vi "Macro Dash.vi"() -> ()   [LabVIEW 2017]
uses:
  VIs/CtrlRefs/GyroTargetInfo.ctl
panel:
  out "CurrentTime":timestamp caption="Robot Time" format="%<%.2X>T"
  in  "Exit":bool
  in  "Tab Control":enum32{"Macro", "Gyro"}(tab)
  out "Boolean":bool
  out "Tank":dbl(slide) caption="Remaining Time" scale=0.0..15.0
  in  "Record Start":bool
  out "Timer":dbl format="%#.1f"
  in  "Record Stop":bool
  in  "Macro Name":string
  in  "Macro delete":bool
  in  "Macros":i32(listbox)
  out "TurnRight":bool
  out "TurnLeft":bool
  out "OnTarget":bool
  out "Gyro":cluster{dbl, dbl}(knob)={0.0, 10.0} scale=0.0..360.0
  # "Tab Controls allow you to have more screens."
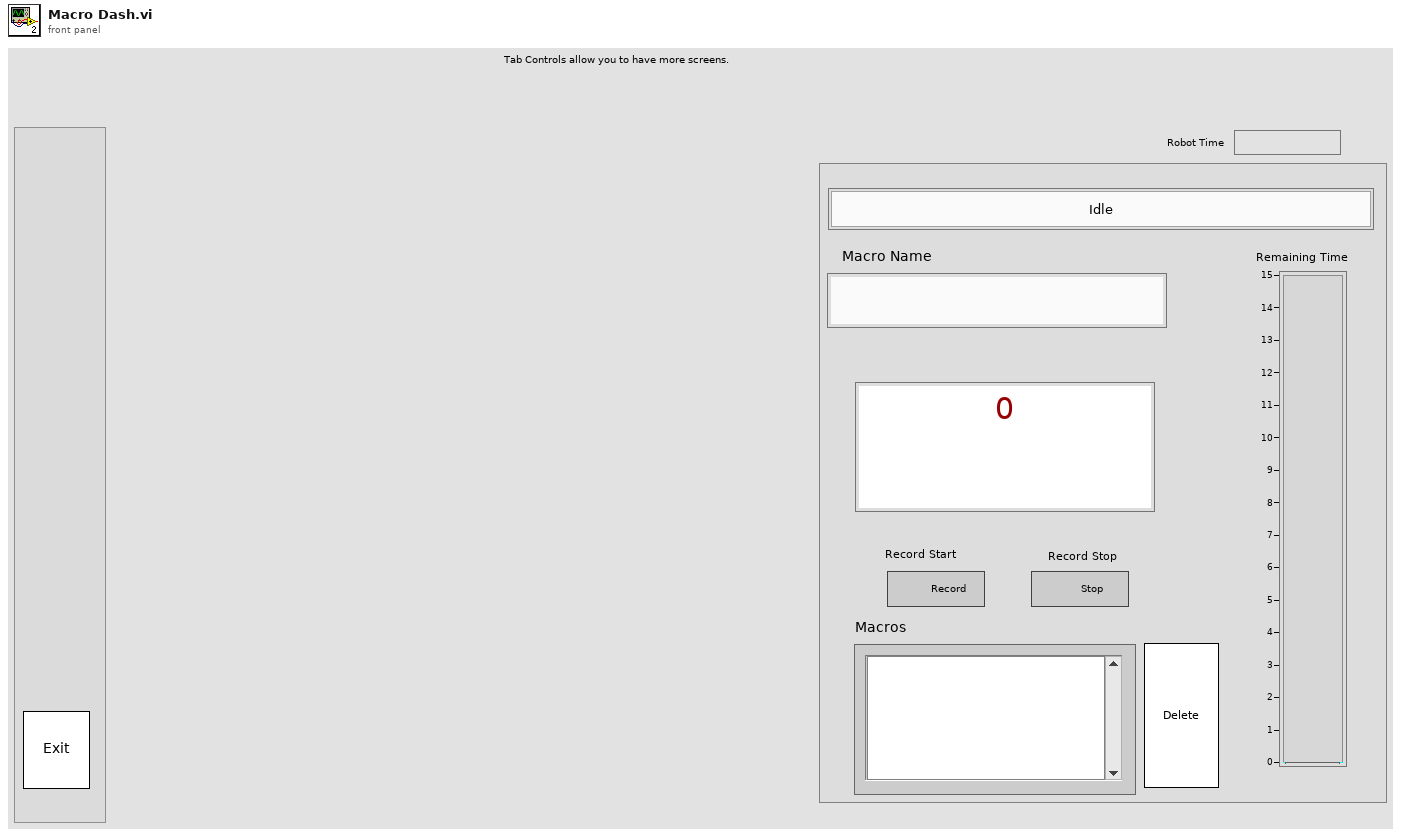
[diagram p1: front panel]
types:
  T1 = typedef "GyroTargetInfo.ctl" = cluster{"Target":dbl, "CurHeading":dbl, "OnTarget":bool, "RotateLeft":bool, "RotateRight":bool, "DegreesToTarget":dbl, "RotDirection":enum16{"Left", "Right", "Stop"}}
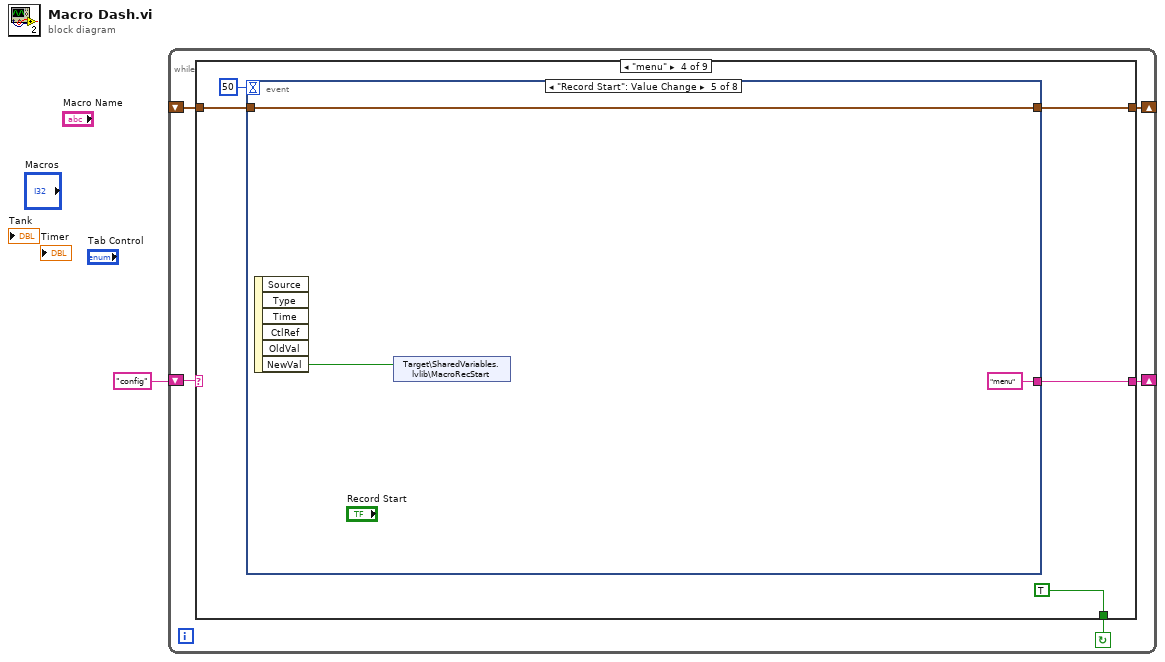
[diagram p0: block diagram]
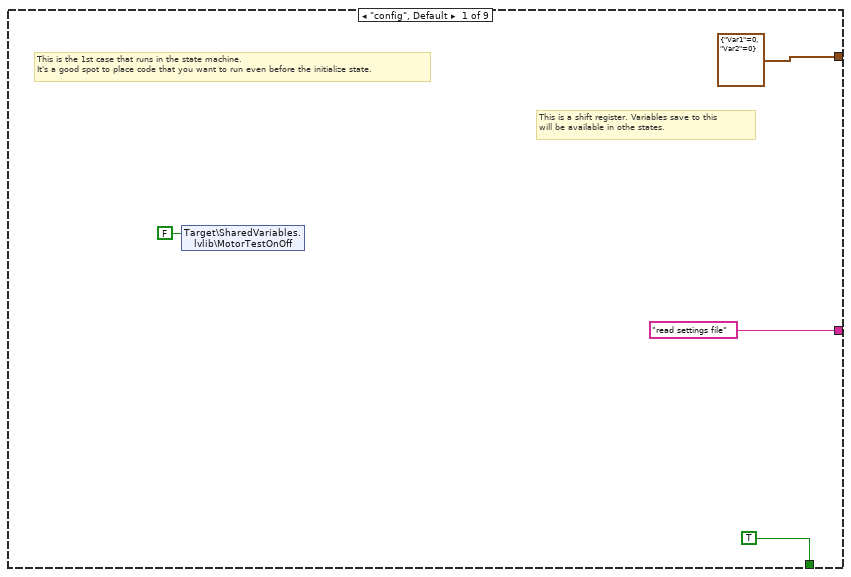
[diagram p2: hidden frame]
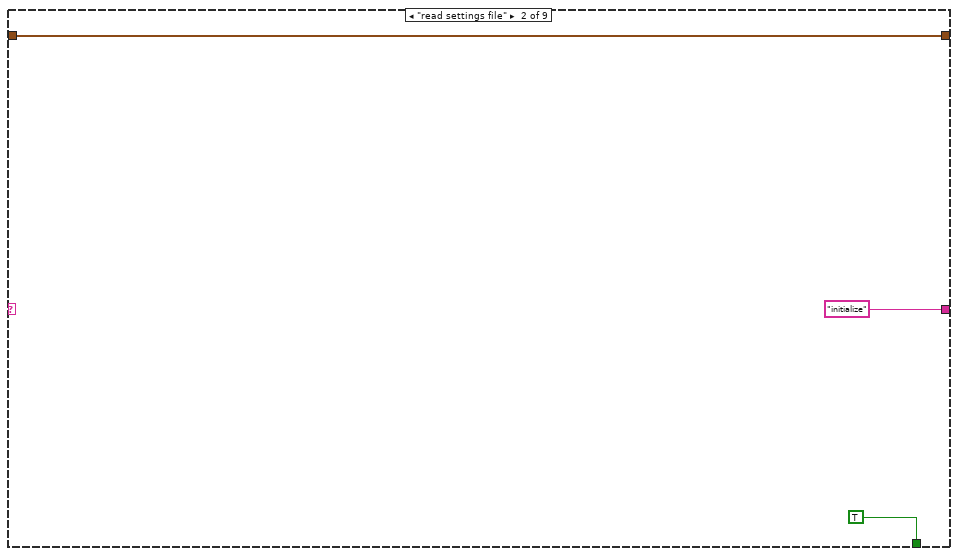
[diagram p3: hidden frame]
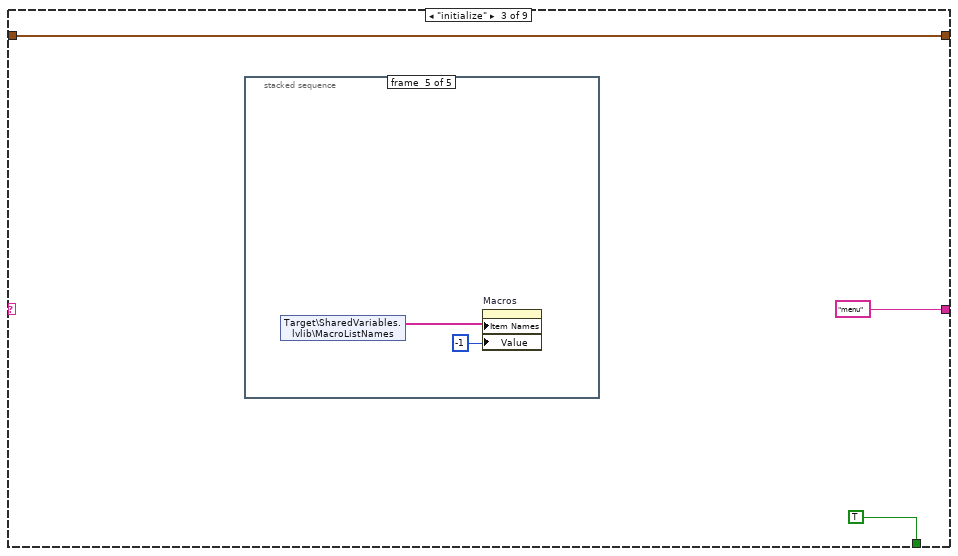
[diagram p4: hidden frame]
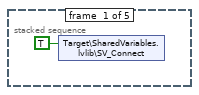
[diagram p5: hidden frame]
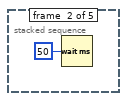
[diagram p6: hidden frame]
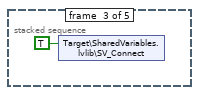
[diagram p7: hidden frame]
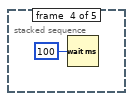
[diagram p8: hidden frame]
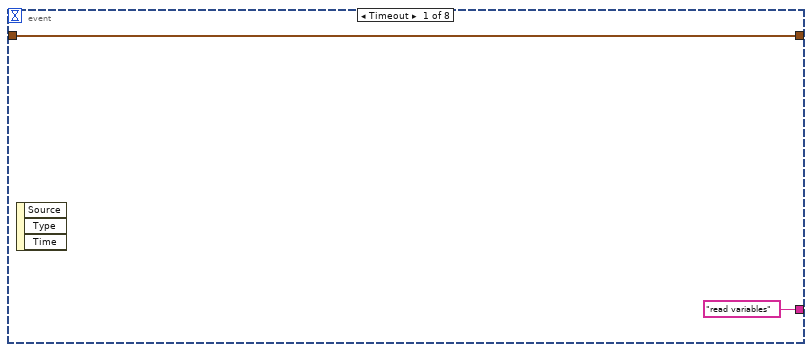
[diagram p9: hidden frame]
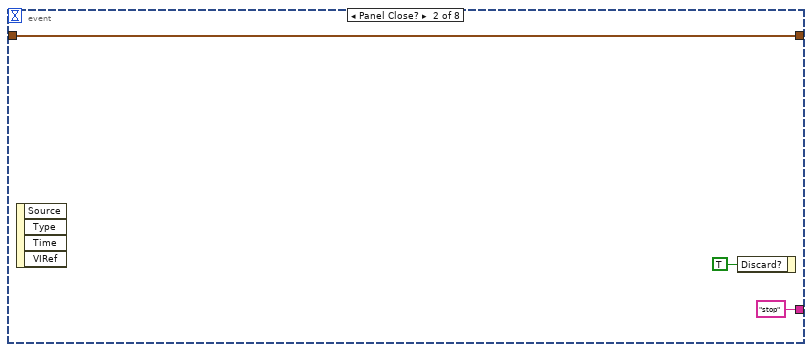
[diagram p10: hidden frame]
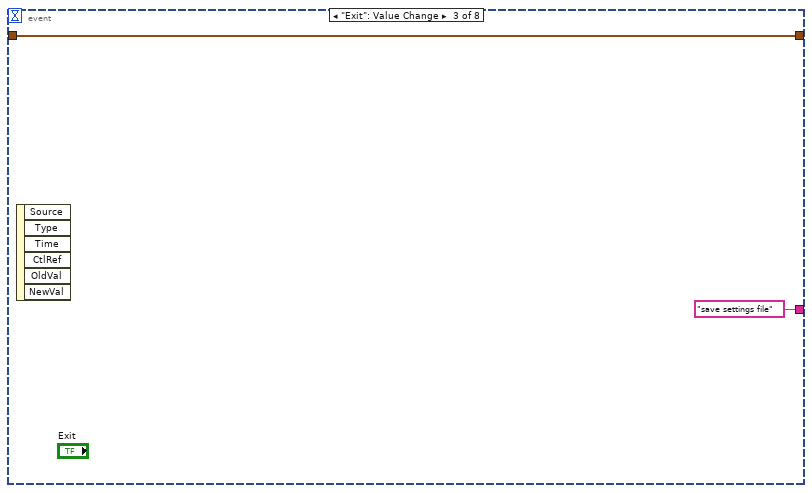
[diagram p11: hidden frame]
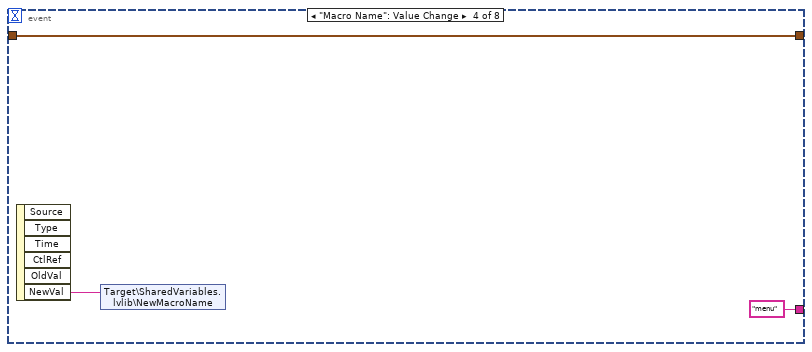
[diagram p12: hidden frame]
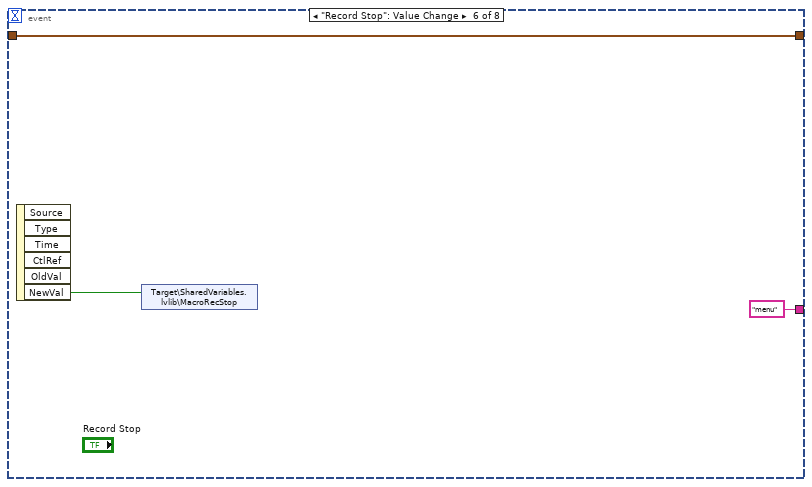
[diagram p13: hidden frame]
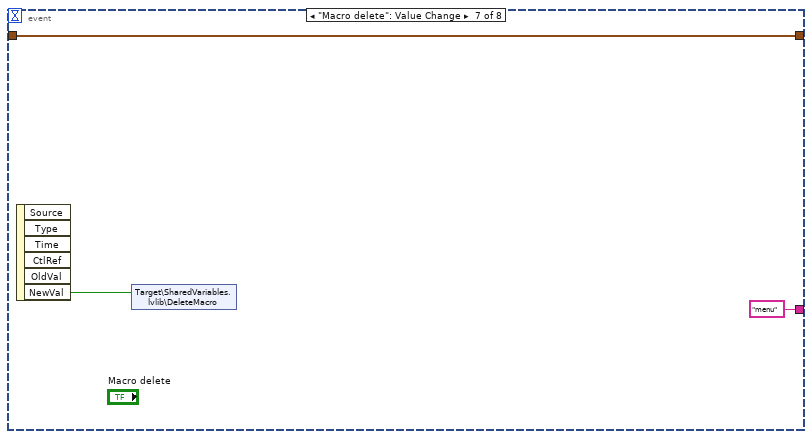
[diagram p14: hidden frame]
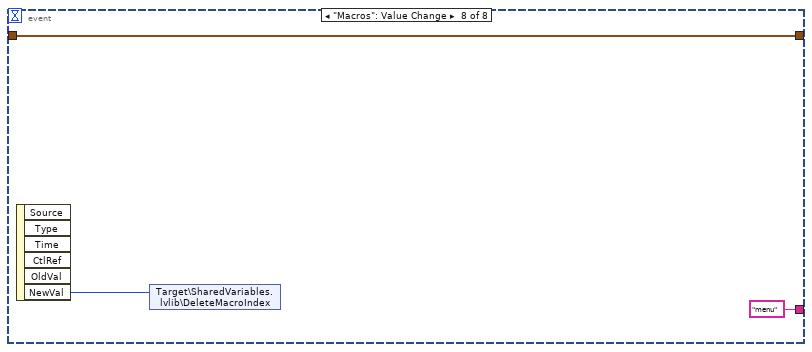
[diagram p15: hidden frame]
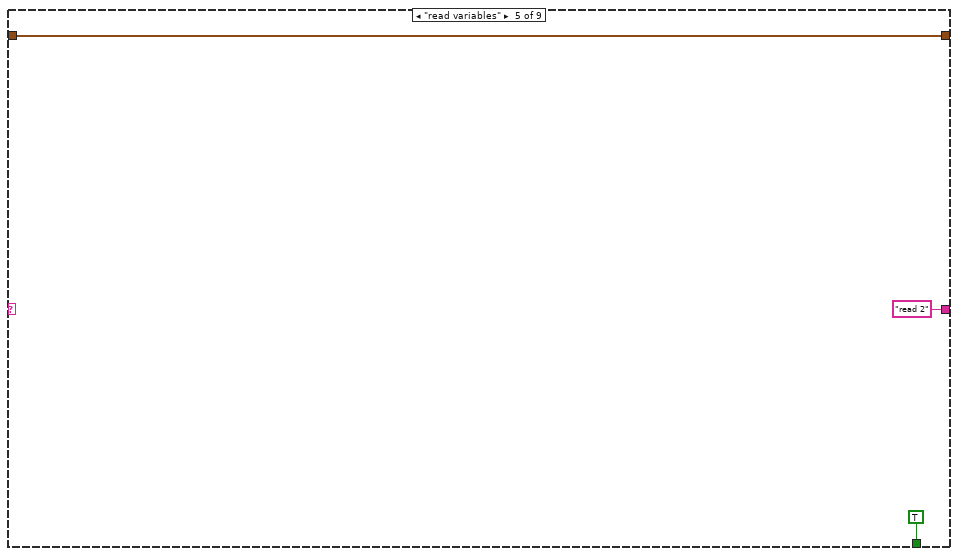
[diagram p16: hidden frame]
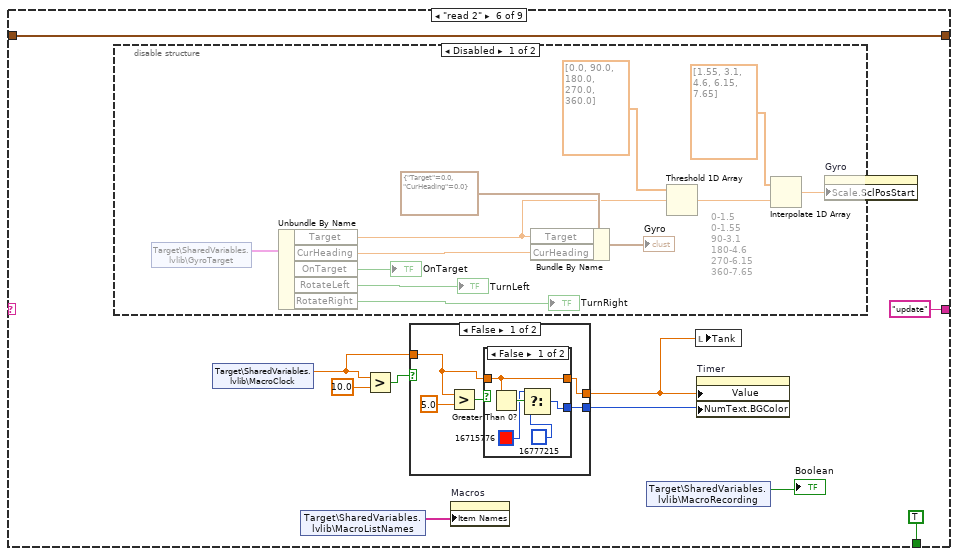
[diagram p17: hidden frame]
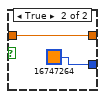
[diagram p19: hidden frame]
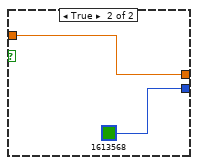
[diagram p20: hidden frame]
diagram:
  n1 = while {
    shift-right: [w4] -> _
    shift-left: "config" -> [w5]
    shift-right: [w3] -> _
    shift-left: _ -> [w2]
    stop <- w6 continue-if-true
    n2 = case shown="\"menu\"" w5 {
      tunnel: [TRUE TRUE TRUE TRUE TRUE TRUE TRUE TRUE FALSE] -> w6
      tunnel: ["read settings file" "initialize" "menu" w26 "read 2" "update" "menu" "stop" "stop"] -> w4
      tunnel: [cluster{"Var1":i32, "Var2":i32} {"Var1"=0, "Var2"=0} w13 w14 w24 w50 w62 w92 w95 w96] -> w3
      tunnel: w2 -> [_ w13 w14 w25 w50 w62 w92 w95 w96]
      frame "config", Default {
        # "This is a shift register. Variables save to this\nwill be available in othe states."
        # "This is the 1st case that runs in the state machine.\nIt's a good spot to place code that you want to run even before the initialize state."
        n3 = shared-variable "Target\\SharedVariables.lvlib\\MotorTestOnOff"(FALSE ("MotorTestOnOff")) -> ()  [unwired: 1 in, 1 out]
      }
      frame "read settings file" {
      }
      frame "initialize" {
        n4 = stacked-sequence {
          frame #0 {
            n5 = shared-variable "Target\\SharedVariables.lvlib\\SV_Connect"(TRUE ("SV_Connect")) -> ()  [unwired: 1 in, 1 out]
          }
          frame #1 {
            n6 = Wait (ms)(milliseconds to wait=u32 50) -> ()  [unwired: 1 out]
          }
          frame #2 {
            n7 = shared-variable "Target\\SharedVariables.lvlib\\SV_Connect"(TRUE ("SV_Connect")) -> ()  [unwired: 1 in, 1 out]
          }
          frame #3 {
            n8 = Wait (ms)(milliseconds to wait=u32 100) -> ()  [unwired: 1 out]
          }
          frame #4 {
            n9 = shared-variable "Target\\SharedVariables.lvlib\\MacroListNames"() -> (w22:string[])  [unwired: 1 in, 1 out]
            n10 = property on="Macros" class="LstBox (strict)"("Item Names"=w22, "Value"=-1 ("Macros")) -> ()  [unwired: 2 in, 2 out]
          }
        }
      }
      frame "menu" {
        n11 = event shown="[4] \"Record Start\": Value Change" {
          selector: _ -> [_ _ _ _ _ _ _ _]
          dyn-events: _ -> [_ _ _ _ _ _ _ _]
          timeout: 50 -> [_ _ _ _ _ _ _ _]
          tunnel: ["read variables" "stop" "save settings file" "menu" "menu" "menu" "menu" "menu"] -> w26
          tunnel: w25 -> [w28 w32 w34 w37 w40 w43 w46 w49]
          tunnel: [w28 w32 w34 w37 w40 w43 w46 w49] -> w24
          event Timeout {
            n12 = event-data() -> ()  [unwired: 1 in, 3 out]
          }
          event Panel Close? {
            n13 = event-data() -> ()  [unwired: 1 in, 4 out]
            n14 = event-data("Discard?"=TRUE) -> ()  [unwired: 1 in, 1 out]
          }
          event "Exit": Value Change {
            n15 = event-data() -> ()  [unwired: 1 in, 6 out]
          }
          event "Macro Name": Value Change {
            n16 = event-data() -> ("NewVal"=w36:string)  [unwired: 1 in, 5 out]
            n17 = shared-variable "Target\\SharedVariables.lvlib\\NewMacroName"(w36) -> ()  [unwired: 1 in, 1 out]
          }
          event "Record Start": Value Change {
            n18 = event-data() -> ("NewVal"=w39:bool)  [unwired: 1 in, 5 out]
            n19 = shared-variable "Target\\SharedVariables.lvlib\\MacroRecStart"(w39) -> ()  [unwired: 1 in, 1 out]
          }
          event "Record Stop": Value Change {
            n20 = event-data() -> ("NewVal"=w42:bool)  [unwired: 1 in, 5 out]
            n21 = shared-variable "Target\\SharedVariables.lvlib\\MacroRecStop"(w42) -> ()  [unwired: 1 in, 1 out]
          }
          event "Macro delete": Value Change {
            n22 = event-data() -> ("NewVal"=w45:bool)  [unwired: 1 in, 5 out]
            n23 = shared-variable "Target\\SharedVariables.lvlib\\DeleteMacro"(w45) -> ()  [unwired: 1 in, 1 out]
          }
          event "Macros": Value Change {
            n24 = event-data() -> ("NewVal"=w48:i32)  [unwired: 1 in, 5 out]
            n25 = shared-variable "Target\\SharedVariables.lvlib\\DeleteMacroIndex"(w48) -> ()  [unwired: 1 in, 1 out]
          }
        }
      }
      frame "read variables" {
      }
      frame "read 2" {
        n26 = disable-structure shown="Disabled" {
          frame Disabled {
            # "0-1.5\n0-1.55\n90-3.1\n180-4.6\n270-6.15\n360-7.65"
            n27 = shared-variable "Target\\SharedVariables.lvlib\\GyroTarget"() -> (w74:T1)  [unwired: 1 in, 1 out]
            n28 = Unbundle By Name(w74) -> ("Target"=w66:dbl, "CurHeading"=w72:dbl, "OnTarget"=→"OnTarget":bool, "RotateLeft"=→"TurnLeft":bool, "RotateRight"=→"TurnRight":bool)
            n29 = Bundle By Name(cluster=cluster{"Target":dbl, "CurHeading":dbl} {"Target"=0.0, "CurHeading"=0.0} ("Gyro"), "Target"=w66, "CurHeading"=w72) -> (→"Gyro":cluster{"Target":dbl, "CurHeading":dbl})
            n30 = Threshold 1D Array(2:w66, 3:dbl[] [0.0, 90.0, 180.0, 270.0, 360.0]) -> (0:w64:dbl)  [unwired: 1 in]
            n31 = Interpolate 1D Array(1:w64, 2:dbl[] [1.55, 3.1, 4.6, 6.15, 7.65]) -> (0:w63:dbl)
            n32 = property on="Gyro" class="Knob (strict)"("Scale.SclPosStart"=w63) -> ()  [unwired: 2 in, 2 out]
          }
          frame Enabled {
          }
        }
        n33 = shared-variable "Target\\SharedVariables.lvlib\\MacroClock"() -> (w55:dbl)  [unwired: 1 in, 1 out]
        n34 = shared-variable "Target\\SharedVariables.lvlib\\MacroListNames"() -> (w59:string[])  [unwired: 1 in, 1 out]
        n35 = Greater?(x=w55, y=10.0) -> (0:w57:bool)
        n36 = case shown="False" w57 {
          tunnel: [w77 u32 1613568] -> w56
          tunnel: w55 -> [w76 w87]
          tunnel: [w75 w87] -> w53
          frame False {
            n37 = Greater?(x=w76, y=5.0) -> (0:w78:bool)
            n38 = case shown="False" w78 {
              tunnel: [w80 u32 16747264] -> w77
              tunnel: w76 -> [w84 w85]
              tunnel: [w84 w85] -> w75
              frame False {
                n39 = Greater Than 0?(x=w84) -> (x > 0?=w83:bool)
                n40 = Select(t=u32 16715776, s=w83, f=u32 16777215) -> (s? t:f=w80:u32)
              }
              frame True {
              }
            }
          }
          frame True {
          }
        }
        n41 = property on="Macros" class="LstBox (strict)"("Item Names"=w59) -> ()  [unwired: 2 in, 2 out]
        n42 = shared-variable "Target\\SharedVariables.lvlib\\MacroRecording"() -> (→"Boolean":bool)  [unwired: 1 in, 1 out]
        n43 = local write "Tank"(w53) -> ()
        n44 = property on="Timer" class="DigNum (strict)"("Value"=w53, "NumText.BGColor"=w56) -> ()  [unwired: 2 in, 2 out]
      }
      frame "update" {
        n45 = shared-variable "Target\\SharedVariables.lvlib\\RoboRioTime"() -> (→"CurrentTime":timestamp)  [unwired: 1 in, 1 out]
      }
      frame "save settings file" {
      }
      frame "stop" {
        n46 = stacked-sequence {
          frame #0 {
            n47 = shared-variable "Target\\SharedVariables.lvlib\\SV_Connect"(FALSE ("SV_Connect")) -> ()  [unwired: 1 in, 1 out]
          }
          frame #1 {
            n48 = Wait (ms)(milliseconds to wait=u32 50) -> ()  [unwired: 1 out]
          }
          frame #2 {
            n49 = shared-variable "Target\\SharedVariables.lvlib\\SV_Connect"(FALSE ("SV_Connect")) -> ()  [unwired: 1 in, 1 out]
          }
          frame #3 {
            # "Only set this to TRUE when making and executable. Otherwise it will close LabVIEW."
            n50 = Quit LabVIEW(quit? (T)=FALSE) -> ()
          }
        }
      }
    }
  }
